vi "Pendulum query Boot.vi"(11 "instance":i32) -> (3 "function return":i32)   [LabVIEW 2014, in "pendulumApp.lvlib"]
doc: "OOTB_API unsigned int Pendulum_queryBoot(int instance);"
uses:
  pendulumApp.lvlib
  pendulumApp.dll
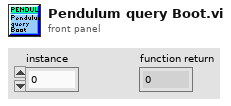
[diagram p1: front panel]
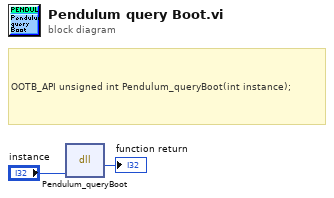
[diagram p0: block diagram]
diagram:
  # "OOTB_API\tunsigned int Pendulum_queryBoot(int instance);"
  n1 = dll-call lib="E:/OneDrive - martint2560@gmail.com/code/SADI_Pendulum/LV/SADI_Pendulum_lib/pendulumApp.*" fn="Pendulum_queryBoot"("instance"="instance") -> ("return type"=→"function return":i32)  [unwired: 4 in, 2 out]
